vi "Save File.vi"(8 "error in (no error)":errorcluster, 10 "Array":string[][](array[string]), 11 "Path":path) -> (0 "error out":errorcluster)   [LabVIEW 2016]
doc: "saves array to csv fspreadsheet file"
uses:
  <vilib>/Utility/file.llb/Write Delimited Spreadsheet (string).vi
  <userlib>/_MGI/File/Spreadsheet/MGI Write Spreadsheet Behavior Enum.ctl
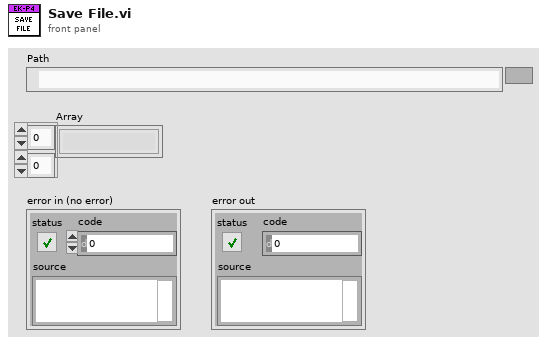
[diagram p1: front panel]
types:
  T1 = typedef "MGI Write Spreadsheet Behavior Enum.ctl" = enum16{"Append data", "Append headers and data", "Overwrite"}
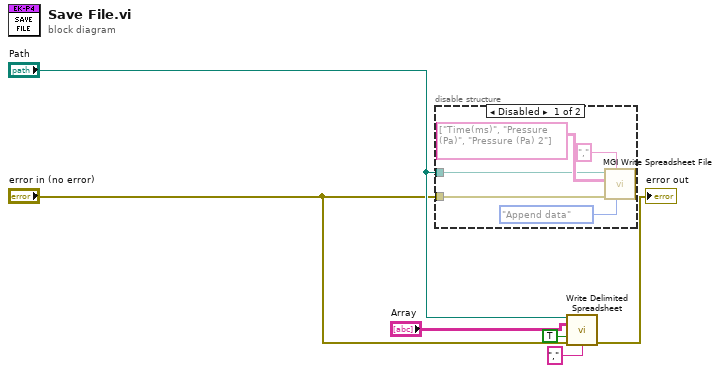
[diagram p0: block diagram]
diagram:
  n1 = disable-structure shown="Disabled" {
    disable-tunnel: "Path" -> [w8 _]
    disable-tunnel: "error in (no error)" -> [w7 _]
    frame Disabled {
      n2 = call <userlib>:"MGI Write Spreadsheet File.vi"("Existing File Behavior"=MGI_Write_Spreadsheet_Behavior_Enum."Append data", "Delimiter (Tab)"=",", "Error In"=w7, "Header Lines[row][col]"=string[][] [["Time(ms)", "Pressure (Pa)", "Pressure (Pa) 2"]], "Path"=w8) -> ()  [unwired: 3 in, 4 out]
    }
    frame Enabled {
    }
  }
  n3 = call-poly <vilib>:"Write Delimited Spreadsheet.vi"("file path (dialog if empty)"="Path", "2D data"="Array", "append to file? (new file:F)"=TRUE, "error in (no error)"="error in (no error)", "delimiter (\\t)"="," ("delimiter (\\t)")) -> ("error out"=→"error out":errorcluster)  [unwired: 9 in, 1 out]
